vi "SetAppStrConstant.vi"(8 "error in (no error)":errorcluster) -> (0 "error out":errorcluster)   [LabVIEW 2020, in "CICD.lvlib"]
doc: "Set constant string in --constant VI to a new value. This VI is used by CICD to update the application name, version and commit SHA based on the current value passed from the automated build pipeline."
uses:
  CICD.lvlib
  <vilib>/Wiresmith Technology/G CLI/CLI Class/CLI.lvclass
  <vilib>/Wiresmith Technology/G CLI/Argument Parser/Option Set Class/Option Set.lvclass
  <vilib>/Wiresmith Technology/G CLI/Argument Parser/Option Class/Option Configuration.ctl
  <vilib>/Wiresmith Technology/G CLI/Argument Parser/Option Class/Option.lvclass
  <vilib>/Wiresmith Technology/G CLI/Argument Parser/Option Class/Argument Type.ctl
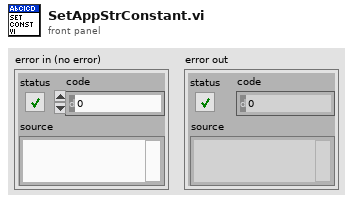
[diagram p1: front panel]
types:
  T1 = typedef "Option Parser.lvlib/Option.lvclass/Option Configuration.ctl" = cluster{"Option Type":T2, "Option Labels":string[], "Key":string, "Description":string, "Required":bool, "Default Value":string}
  T2 = typedef "Option Parser.lvlib/Option.lvclass/Argument Type.ctl" = enum16{"flag", "value"}
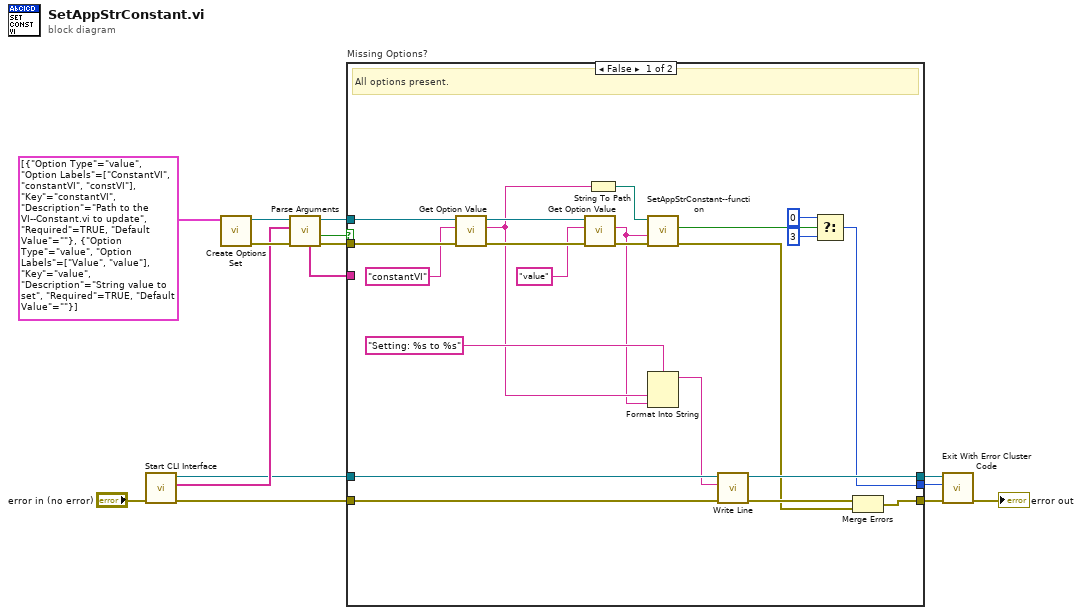
[diagram p0: block diagram]
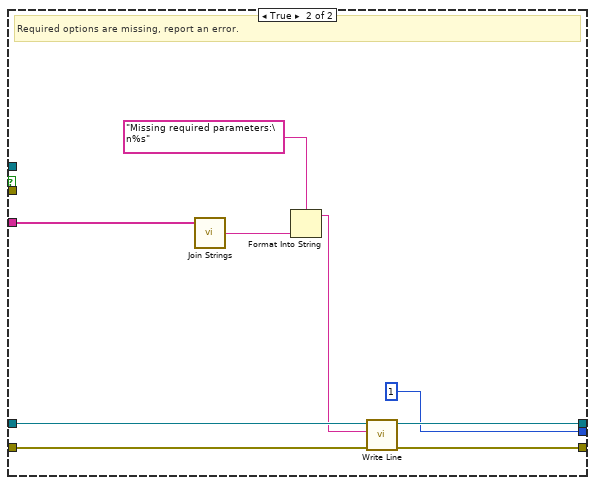
[diagram p2: hidden frame]
diagram:
  n1 = call <vilib>:"Start CLI Interface.vi"("error in (no error)"="error in (no error)") -> ("error out"=w7:errorcluster, "Custom Parameters"=w11:string[], "CLI out"=w6:refnum<class "CLI.lvclass">)  [unwired: 7 in, 1 out]
  n2 = call <vilib>:"Create Options Set.vi"("Options"=T1[] [{"Option Type"=enum."value", "Option Labels"=["ConstantVI", "constantVI", "constVI"], "Key"="constantVI", "Description"="Path to the VI--Constant.vi to update", "Required"=TRUE, "Default Value"=""}, {"Option Type"=enum."value", "Option Labels"=["Value", "value"], "Key"="value", "Description"="String value to set", "Required"=TRUE, "Default Value"=""}]) -> ("error out"=w13:errorcluster, "Option Set out"=w14:refnum<class "Option Set.lvclass">)  [unwired: 9 in]
  n3 = call <vilib>:"Parse Arguments.vi"("error in (no error)"=w13, "Arguments"=w11, "Option Set in"=w14) -> ("error out"=w9:errorcluster, "Missing Options"=w10:bool, "Option Set out"=w1:refnum<class "Option Set.lvclass">, "Missing Option Keys"=w8:string[])  [unwired: 5 in]
  n4 = case "Missing Options?" shown="False" w10 {
    tunnel: w9 -> [w36 _]
    tunnel: w8 -> [_ w44]
    tunnel: w7 -> [w37 w43]
    tunnel: w6 -> [w32 w42]
    tunnel: [w30 w40] -> w5
    tunnel: [w31 w39] -> w3
    tunnel: [w17 1 ("No Error Code (0)")] -> w2
    tunnel: w1 -> [w35 _]
    frame False {
      # "All options present."
      n5 = call <vilib>:"Get Option Value.vi"("error in (no error)"=w36, "Option Key"="constantVI", "Option Set in"=w35) -> ("error out"=w27:errorcluster, "Value"=w24:string, "Option Set out"=w26:refnum<class "Option Set.lvclass">)  [unwired: 5 in, 1 out]
      n6 = call <vilib>:"Get Option Value.vi"("error in (no error)"=w27, "Option Key"="value", "Option Set in"=w26) -> ("error out"=w22:errorcluster, "Value"=w16:string)  [unwired: 5 in, 2 out]
      n7 = String To Path(string=w24) -> (path=w23:path)
      n8 = call "SetAppStrConstant--function.vi"("error in"=w22, "Value"=w16, "vi path"=w23) -> ("error out"=w20:errorcluster, "found?"=w21:bool)  [unwired: 7 in]
      n9 = Format Into String(format string="Setting: %s to %s", w24, w16) -> (resulting string=w28:string)  [unwired: 2 in, 1 out]
      n10 = call <vilib>:"Write Line.vi"("error in (no error)"=w37, "Text to Write"=w28, "CLI in"=w32) -> ("error out"=w33:errorcluster, "CLI out"=w31:refnum<class "CLI.lvclass">)  [unwired: 7 in]
      n11 = Select(t=0, s=w21, f=3) -> (s? t:f=w17:i32)
      n12 = Merge Errors(w33, w20) -> (w30:errorcluster)
    }
    frame True {
      # "Required options are missing, report an error."
      n13 = call <vilib>:"Join Strings.vi"("Strings In"=w44) -> ("String"=w45:string)  [unwired: 2 in]
      n14 = Format Into String(format string="Missing required parameters:\n%s" ("Text to Write"), w45) -> (resulting string=w41:string)  [unwired: 2 in, 1 out]
      n15 = call <vilib>:"Write Line.vi"("error in (no error)"=w43, "Text to Write"=w41, "CLI in"=w42) -> ("error out"=w40:errorcluster, "CLI out"=w39:refnum<class "CLI.lvclass">)  [unwired: 7 in]
    }
  }
  n16 = call <vilib>:"Exit With Error Cluster Code.vi"("error in (no error)"=w5, "No Error Code (0)"=w2, "CLI in"=w3) -> ("error out"=→"error out":errorcluster)  [unwired: 8 in]
